vi "Litho Interpolater.vi"(1 "Lithography Data In":T2(array[cluster]), 2 "Distance":dbl) -> (0 "Lithography Data Out":T1(array[cluster]))   [LabVIEW 2011]
doc: "This VI takes lithography information as an input and interpolates points between and within patterns. It also maps voltages onto colors for the simulator."
uses:
  AFM Simulation/Global Variables.vi
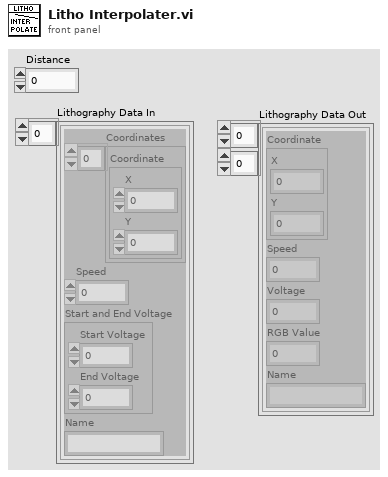
[diagram p1: front panel]
types:
  T1 = cluster{"Coordinate":cluster{"X":dbl, "Y":dbl}, "Speed":dbl, "Voltage":dbl, "RGB Value":i32, "Name":string}[][]
  T2 = cluster{"Coordinates":cluster{"X":dbl, "Y":dbl}[], "Speed":dbl, "Start and End Voltage":cluster{"Start Voltage":dbl, "End Voltage":dbl}, "Name":string}[]
  T3 = cluster{"Coordinate":cluster{"X":dbl, "Y":dbl}, "Speed":dbl, "Voltage":dbl, "index":i32, "Name":string}
  T4 = cluster{"Point cordinate":cluster{"X":dbl, "Y":dbl}, "Speed":dbl, dbl, i32, "Name":string}
  T5 = cluster{"Point cordinate":cluster{"X":dbl, "Y":dbl}, "Speed":dbl, "Voltage":dbl, "index":i32, "Name":string}[]
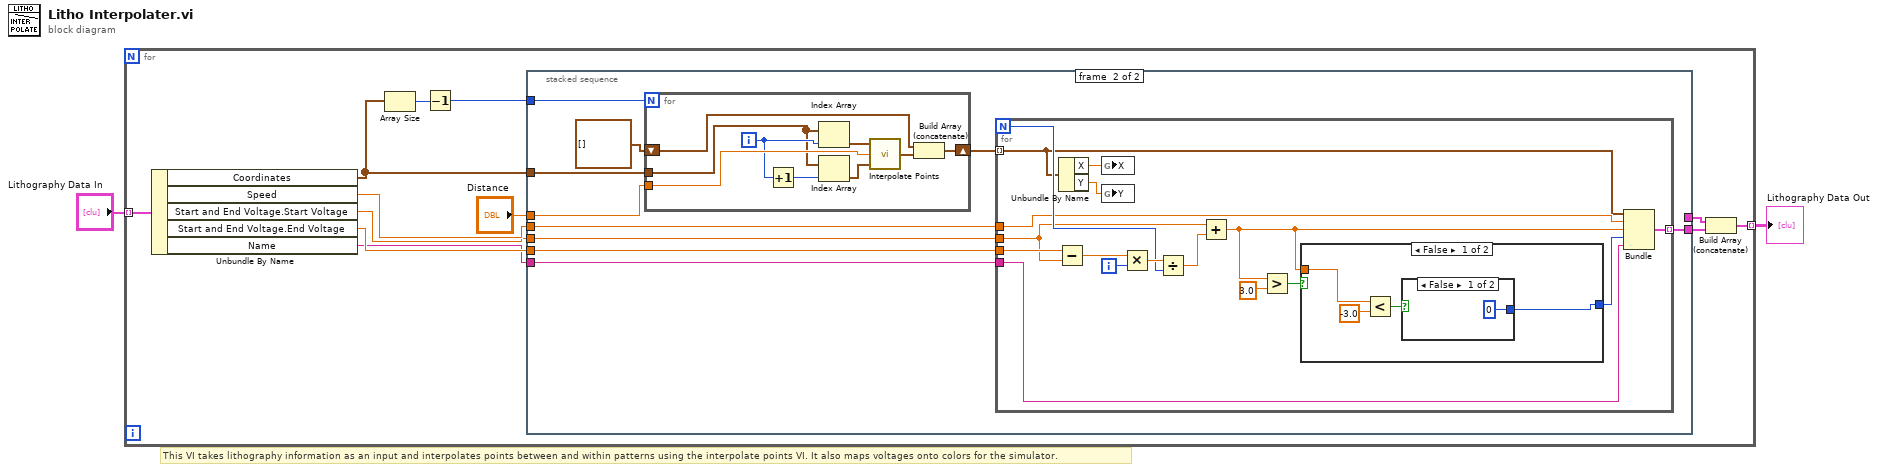
[diagram p0: block diagram]
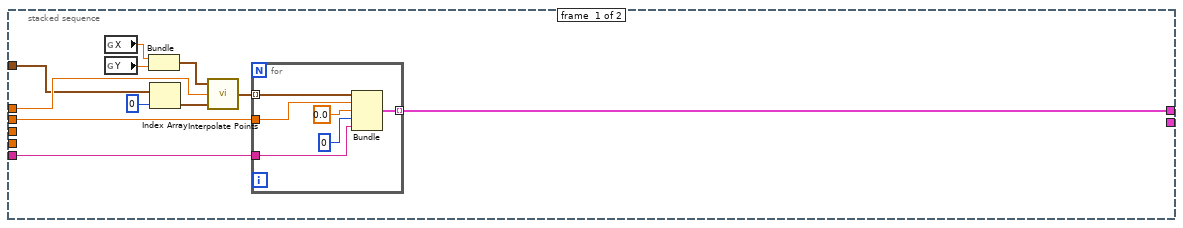
[diagram p2: hidden frame]
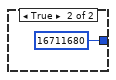
[diagram p3: hidden frame]
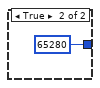
[diagram p4: hidden frame]
diagram:
  # "This VI takes lithography information as an input and interpolates points between and within patterns using the interpolate points VI. It also maps voltages onto colors for the simulator."
  n1 = for {
    tunnel: "Lithography Data In" -> [w14] mode=indexing
    tunnel: [w5] -> w1 mode=indexing
    n2 = Unbundle By Name(w14) -> ("Coordinates"=w11:cluster{"X":dbl, "Y":dbl}[], "Speed"=w10:dbl, "Start and End Voltage.Start Voltage"=w9:dbl, "Start and End Voltage.End Voltage"=w8:dbl, "Name"=w4:string)
    n3 = Array Size(array=w11) -> (size(s)=w13:i32)
    n4 = Decrement(x=w13) -> (x-1=w12:i32)
    n5 = stacked-sequence {
      tunnel: "Distance" -> [w25 w41]
      tunnel: w12 -> [_ w40]
      tunnel: w11 -> [w24 w39]
      tunnel: w10 -> [w17 w38]
      tunnel: w9 -> [_ w37]
      tunnel: w8 -> [_ w36]
      tunnel: [w16 _] -> w7
      tunnel: [_ w33] -> w6
      tunnel: w4 -> [w15 w32]
      frame #0 {
        n6 = global read "Global Variables.vi" "X"() -> (w20:dbl)
        n7 = global read "Global Variables.vi" "Y"() -> (w21:dbl)
        n8 = Bundle("X"=w20, "Y"=w21) -> (w19:cluster{"X":dbl, "Y":dbl})  [unwired: 1 in]
        n9 = Index Array(array=w24, index=0) -> (element=w22:cluster{"X":dbl, "Y":dbl})
        n10 = call "Interpolate Points.vi"("End Point"=w22, "Distance between Points"=w25, "Start Point"=w19) -> ("Output Point Array"=w18:cluster{"X":dbl, "Y":dbl}[])
        n11 = for {
          tunnel: w18 -> [w31] mode=indexing
          tunnel: w17 -> [w30]
          tunnel: [w28] -> w16 mode=indexing
          tunnel: w15 -> [w26]
          n12 = Bundle("Coordinate"=w31, "Speed"=w30, "Voltage"=0.0, "index"=0, "Name"=w26) -> (w28:T3)  [unwired: 1 in]
        }
      }
      frame #1 {
        n13 = for {
          N: w40 -> [_]
          tunnel: w41 -> [w74]
          tunnel: w39 -> [w71]
          shift-right: [w66] -> w34
          shift-left: cluster{"X":dbl, "Y":dbl}[] [] ("array") -> [w67]
          i -> [w73]
          n14 = Increment(x=w73) -> (x+1=w72:i32)
          n15 = Index Array(array=w71, index=w73) -> (element=w69:cluster{"X":dbl, "Y":dbl})
          n16 = Index Array(array=w71, index=w72) -> (element=w70:cluster{"X":dbl, "Y":dbl})
          n17 = call "Interpolate Points.vi"("End Point"=w70, "Distance between Points"=w74, "Start Point"=w69) -> ("Output Point Array"=w68:cluster{"X":dbl, "Y":dbl}[])
          n18 = Build Array (concatenate)(w67, w68) -> (w66:cluster{"X":dbl, "Y":dbl}[])
        }
        n19 = for {
          N -> [w54]
          tunnel: w34 -> [w51] mode=indexing
          tunnel: w38 -> [w53]
          tunnel: w37 -> [w47]
          tunnel: w36 -> [w58]
          tunnel: [w52] -> w33 mode=indexing
          tunnel: w32 -> [w42]
          i -> [w56]
          n20 = Subtract(x=w58, y=w47) -> (x-y=w57:dbl)
          n21 = Unbundle By Name(w51) -> ("X"=w50:dbl, "Y"=w49:dbl)
          n22 = global write "Global Variables.vi" "X"(w50) -> ()
          n23 = global write "Global Variables.vi" "Y"(w49) -> ()
          n24 = Multiply(x=w57, y=w56) -> (x*y=w55:dbl)
          n25 = Divide(x=w55, y=w54) -> (x/y=w48:dbl)
          n26 = Add(x=w47, y=w48) -> (x+y=w43:dbl)
          n27 = Greater?(x=w43, y=3.0) -> (0:w45:bool)
          n28 = case shown="False" w45 {
            tunnel: [w62 65280] -> w44
            tunnel: w43 -> [w60 _]
            frame False {
              n29 = Less?(x=w60, y=-3.0) -> (x < y?=w59:bool)
              n30 = case shown="False" w59 {
                tunnel: [0 16711680] -> w62
                frame False {
                }
                frame True {
                }
              }
            }
            frame True {
            }
          }
          n31 = Bundle("Point cordinate"=w51, "Speed"=w53, w43, w44, "Name"=w42) -> (w52:T4)  [unwired: 1 in]
        }
      }
    }
    n32 = Build Array (concatenate)(w7, w6) -> (w5:T5)
  }
  "Lithography Data Out" <- w1
